vi "Message Display.vi"(9 "Display Time":u32=1000, 11 "Input Message":string) -> ()   [LabVIEW 2024]
uses:
  USER32.DLL
panel:
  out "String":string
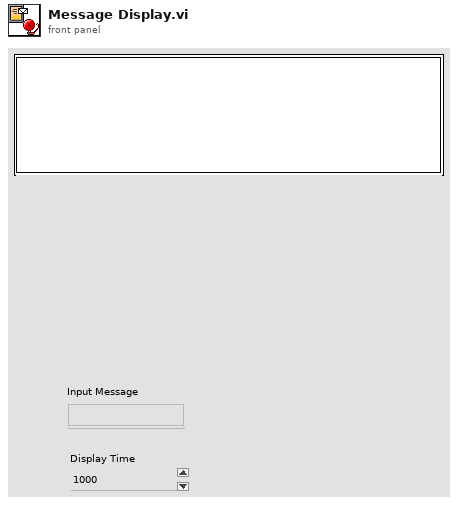
[diagram p1: front panel]
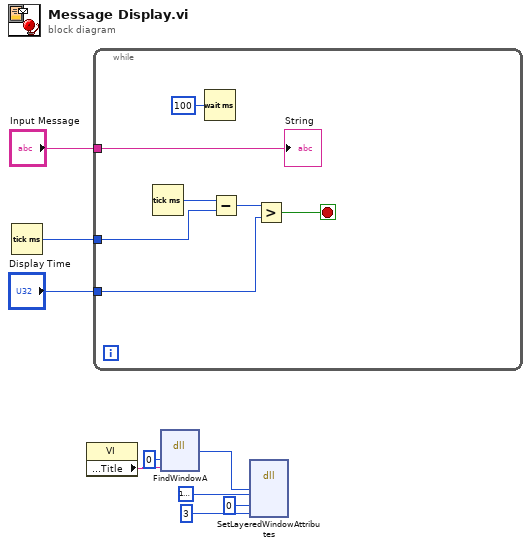
[diagram p0: block diagram]
diagram:
  n1 = Tick Count (ms)() -> (millisecond timer value=w9:u32)
  n2 = property class="VI"() -> ("Front Panel Window:Title"=w6:string)  [unwired: 2 in, 2 out]
  n3 = while {
    tunnel: w9 -> [w14]
    tunnel: "Input Message" -> [w12]
    tunnel: "Display Time" -> [w11]
    stop <- w10 stop-if-true
    n4 = Tick Count (ms)() -> (millisecond timer value=w15:u32)
    n5 = Wait (ms)(milliseconds to wait=u32 100) -> ()  [unwired: 1 out]
    n6 = Subtract(x=w15, y=w14) -> (x-y=w13:u32)
    n7 = Greater?(x=w13, y=w11) -> (0:w10:bool)
    "String" <- w12
  }
  n8 = dll-call lib="User32.dll" fn="FindWindowA" label="FindWindow"("lpszClassName"=0, w6) -> ("hWnd"=w4:u16)  [unwired: 5 in, 2 out]
  n9 = dll-call lib="USER32.DLL" fn="SetLayeredWindowAttributes" label="SetLayerdWindowAttributs"("handle"=w4, "crkey"=u32 16777216, "bAlpha"=0, "dwFlags"=3) -> ()  [unwired: 8 in, 2 out]
